vi "oa_Search Start and End in Speed Profile (time).vi"(6 "last value in":cluster{"reference":dbl, "interpolation":dbl}, 7 "reset":bool, 8 "steps input":cluster{"start":dbl, "end":dbl, "step":dbl} {"step" format="%.2f"; "end" format="%.2f"; "start" format="%.2f"}, 9 "next value in":dbl, 10 "interpolation array":dbl[](array[numeric]), 11 "reference array":dbl[](array[numeric])) -> (0 "actual steps":T1 {"step" format="%.2f"; "start" format="%.2f"}, 1 "next value out":dbl, 2 "interpolation array out":dbl[](array[numeric]), 3 "reference array out":dbl[](array[numeric]), 4 "last value out":cluster{"reference":dbl, "interpolation":dbl}, 5 "reach end?":bool)   [LabVIEW 2017]
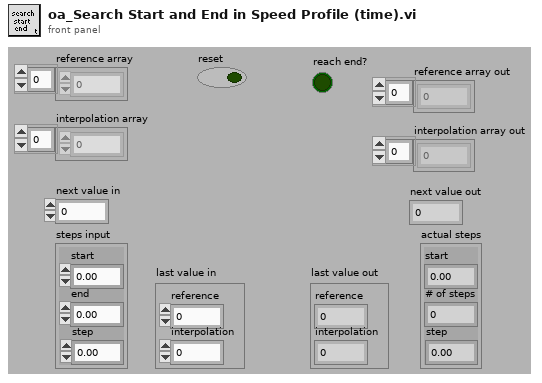
[diagram p1: front panel]
types:
  T1 = cluster{"start":dbl, "# of steps":i32, "step":dbl}
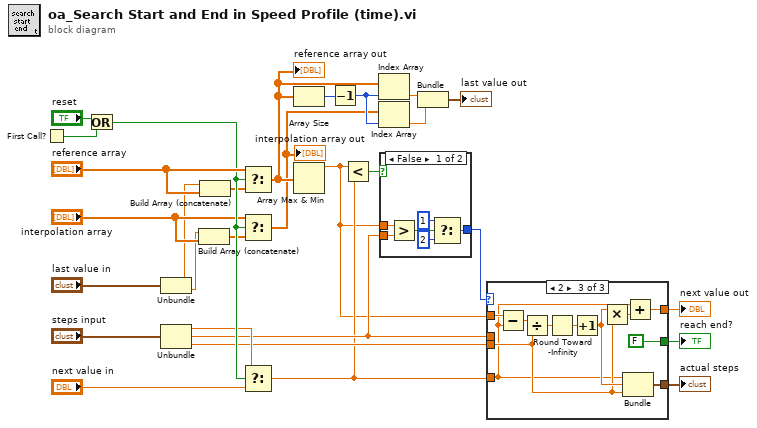
[diagram p0: block diagram]
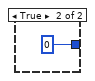
[diagram p2: hidden frame]
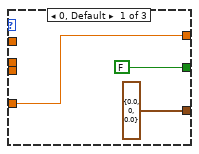
[diagram p3: hidden frame]
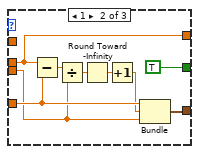
[diagram p4: hidden frame]
diagram:
  n1 = First Call?() -> (First Call?: T/F=w27:bool)
  n2 = Or(x="reset", y=w27) -> (x .or. y?=w23:bool)
  n3 = Unbundle("last value in") -> ("reference"=w17:dbl, "interpolation"=w14:dbl)
  n4 = Unbundle("steps input") -> ("start"=w18:dbl, "end"=w8:dbl, "step"=w7:dbl)
  n5 = Build Array (concatenate)(w14, "interpolation array") -> (w15:dbl[])
  n6 = Build Array (concatenate)(w17, "reference array") -> (w16:dbl[])
  n7 = Select(t="reference array", s=w23, f=w16) -> (s? t:f=w6:dbl[])
  "reference array out" <- w6
  n8 = Select(t="interpolation array", s=w23, f=w15) -> (s? t:f=w5:dbl[])
  "interpolation array out" <- w5
  n9 = Select(t=w18, s=w23, f="next value in") -> (s? t:f=w3:dbl)
  n10 = Array Size(array=w6) -> (size(s)=w13:i32)
  n11 = Array Max & Min(array=w6) -> (max value=w2:dbl)  [unwired: 3 out]
  n12 = Decrement(x=w13) -> (x-1=w12:i32)
  n13 = Less?(x=w2, y=w3) -> (x < y?=w1:bool)
  n14 = Index Array(array=w6, index=w12) -> (element=w11:dbl)
  n15 = Index Array(array=w5, index=w12) -> (element=w10:dbl)
  n16 = case shown="False" w1 {
    tunnel: w2 -> [w35 _]
    tunnel: w8 -> [w34 _]
    tunnel: [w30 0] -> w4
    frame False {
      n17 = Greater?(x=w35, y=w34) -> (0:w33:bool)
      n18 = Select(t=1, s=w33, f=2) -> (s? t:f=w30:i32)
    }
    frame True {
    }
  }
  n19 = Bundle("time [s]"=w11, "speed [rpm]"=w10) -> (→"last value out":cluster{"time [s]":dbl, "speed [rpm]":dbl})  [unwired: 1 in]
  n20 = case shown="2" w4 {
    tunnel: [FALSE ("reach end?") TRUE ("reach end?") FALSE ("reach end?")] -> w21
    tunnel: w3 -> [w38 w47 w51]
    tunnel: [w38 w42 w53] -> w20
    tunnel: [T1 {"start"=0.0, "# of steps"=0, "step"=0.0} ("actual steps") w43 w57] -> w19
    tunnel: w7 -> [_ w45 w55]
    tunnel: w8 -> [_ w42 _]
    tunnel: w2 -> [_ _ w52]
    frame 0, Default {
    }
    frame 1 {
      n21 = Subtract(x=w42, y=w47) -> (x-y=w46:dbl)
      n22 = Divide(x=w46, y=w45) -> (x/y=w41:dbl)
      n23 = Round Toward -Infinity(1:w41) -> (0:w40:dbl)
      n24 = Increment(x=w40) -> (x+1=w44:dbl)
      n25 = Bundle("next value in"=w47, w44, "step"=w45) -> (w43:cluster{"next value in":dbl, dbl, "step":dbl})  [unwired: 1 in]
    }
    frame 2 {
      n26 = Subtract(x=w52, y=w51) -> (x-y=w58:dbl)
      n27 = Divide(x=w58, y=w55) -> (x/y=w50:dbl)
      n28 = Round Toward -Infinity(1:w50) -> (0:w49:dbl)
      n29 = Increment(x=w49) -> (x+1=w56:dbl)
      n30 = Multiply(x=w56, y=w55) -> (x*y=w54:dbl)
      n31 = Bundle("next value in"=w51, w56, "step"=w55) -> (w57:cluster{"next value in":dbl, dbl, "step":dbl})  [unwired: 1 in]
      n32 = Add(x=w51, y=w54) -> (x+y=w53:dbl)
    }
  }
  "next value out" <- w20
  "reach end?" <- w21
  "actual steps" <- w19
